vi "clFileReader_readInt.vi"(9 "size":u32=4, 10 "offset":u32, 11 "clFileReader.lvclass IN":refnum<class "clFileReader.lvclass">) -> (0 "OUT Value":u32, 1 "EOF?":bool, 2 "new offset":u32, 3 "clFileReader.lvclass OUT":refnum<class "clFileReader.lvclass">)   [LabVIEW 2021, in "vi_lib.lvlib" / "clFileReader.lvclass"]
uses:
  clFileReader.lvclass
  clFileReader.lvclass/clFileReader.ctl
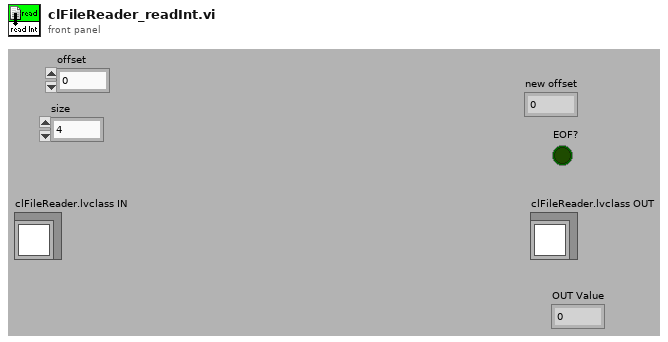
[diagram p1: front panel]
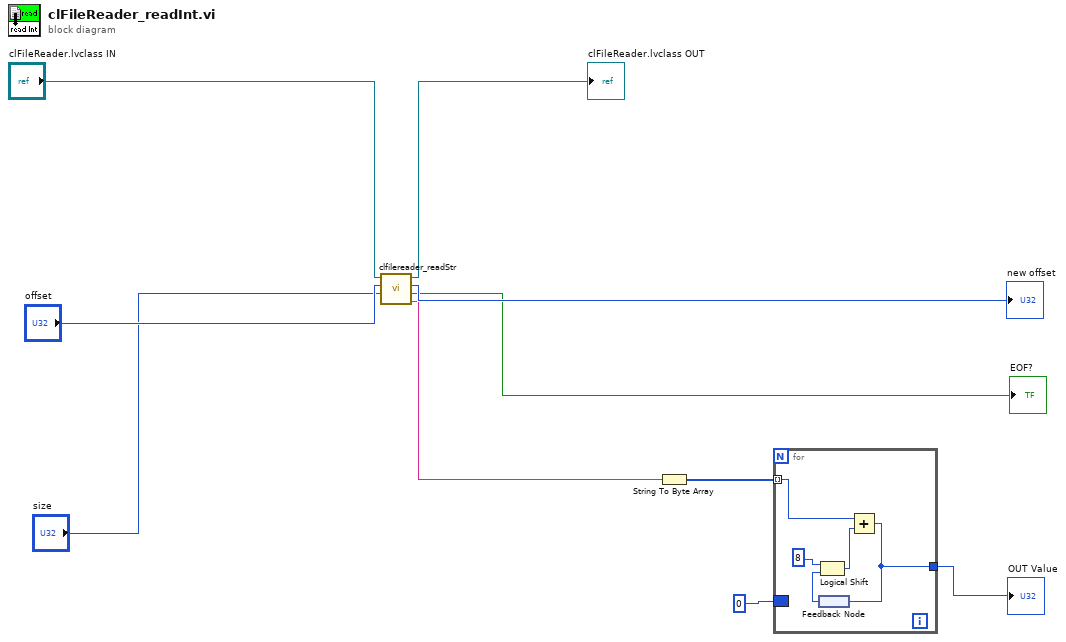
[diagram p0: block diagram]
diagram:
  n1 = call "clfilereader_readStr.vi"("size"="size", "offset"="offset", "clFileReader.lvclass IN"="clFileReader.lvclass IN") -> ("ReadStr - OUT Value"=w4:string, "EOF?"=→"EOF?":bool, "new offset"=→"new offset":u32, "clFileReader.lvclass OUT"=→"clFileReader.lvclass OUT":refnum<class "clFileReader.lvclass">)  [unwired: 5 out]
  n2 = String To Byte Array(string=w4) -> (unsigned byte array=w3:u8[])
  n3 = for {
    tunnel: w3 -> [w15] mode=indexing
    border: 0 -> [_]
    tunnel: [w13] -> w1
    n4 = feedback #1() -> (w12:i32)
    n5 = Logical Shift(y=8 ("x"), x=w12) -> (x << y=w14:i32)
    n6 = Add(x=w15, y=w14) -> (x+y=w13:i32)
    n7 = feedback-in #1(w13) -> ()
  }
  "OUT Value" <- w1
